vi "Iterate.vi"(6 "notifier in":refnum<notifier>, 8 "error in (no error)":errorcluster, 10 "Iterator Settings":T1={"Prepare timeout (ms)"=200, "Iterate timeout (ms)"=50, "Conclude timeout (ms)"=200, "Iterate period (ms)"=200, "Number of iterations"=5, "Stop Condition"=enum."None", "Time before stop (ms)"=5, "Prepare Msg"=refnum, "Iterate Msg"=refnum, "Conclude Msg"=refnum, "Error Handler"=refnum}, 11 "Caller Enqueuer in":refnum<class "Message Enqueuer.lvclass">) -> (0 "error out":errorcluster, 3 "Caller Enqueuer out":refnum<class "Message Enqueuer.lvclass">)   [LabVIEW 2017, in "Iterator Actor.lvlib" / "Iterator Actor.lvclass"]
doc: "Iteratively calls the Iterate method of the Client. \nStops the iterations either by receiving the Stop signal, or by any of predefined Stop conditions."
uses:
  Iterator Actor.lvclass
  Iterator Settings.ctl
  Iterator Actor Abstract Messages/Iterator Reply Msg/Iterator Reply Msg.lvclass
  C:/Program Files (x86)/National Instruments/LabVIEW 2017/vi.lib/ActorFramework/Message/Message.lvclass
  Iterator Actor Abstract Messages/Iterator Report Error Msg/Iterator Report Error Msg.lvclass
  Stop Condition.ctl
  <vilib>/ActorFramework/Message Enqueuer/Message Enqueuer.lvclass
  Iterator Actor Abstract Messages/Iterator Reply Msg/Iterator Reply Msg.lvclass/Iterator Reply Msg.ctl
  <vilib>/ActorFramework/Message Enqueuer/Message Enqueuer.lvclass/Message Enqueuer.ctl
  Iterator Errors.ctl
  <vilib>/ActorFramework/Message Enqueuer/Enqueue.vi
  <vilib>/ActorFramework/Message Priority Queue/Priority Enqueue.vi
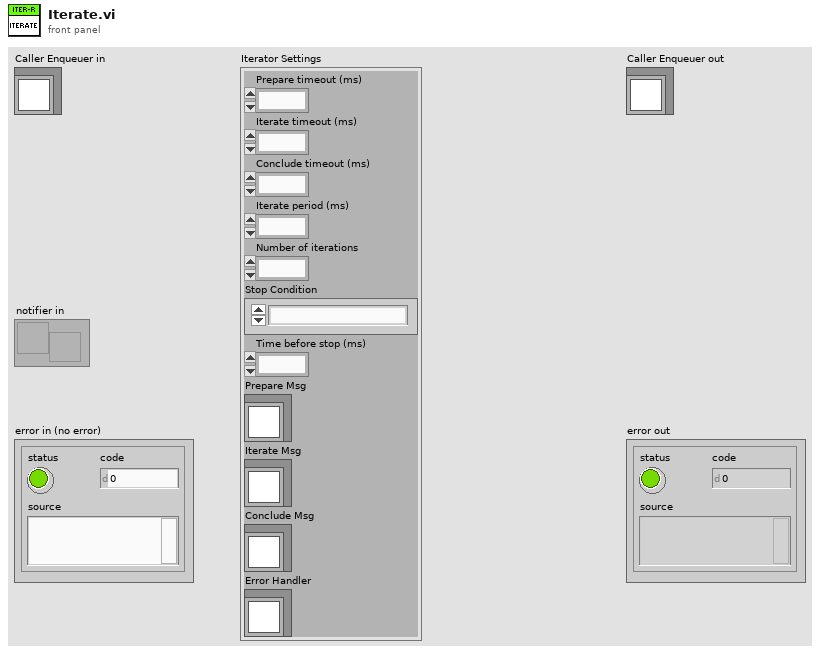
[diagram p1: front panel]
types:
  T1 = typedef "Iterator Actor.lvlib/Iterator Actor.lvclass/Iterator Settings.ctl" = cluster{"Prepare timeout (ms)":i32, "Iterate timeout (ms)":i32, "Conclude timeout (ms)":i32, "Iterate period (ms)":i32, "Number of iterations":i32, "Stop Condition":T2, "Time before stop (ms)":i32, "Prepare Msg":refnum<class "Iterator Reply Msg.lvclass">, "Iterate Msg":refnum<class "Iterator Reply Msg.lvclass">, "Conclude Msg":refnum<class "Iterator Reply Msg.lvclass">, "Error Handler":refnum<class "Iterator Report Error Msg.lvclass">}
  T2 = typedef "Iterator Actor.lvlib/Iterator Actor.lvclass/Stop Condition.ctl" = enum16{"None", "Number of Iterations", "Time Elapsed", "Iteration Result"}
  T3 = typedef "Iterator Actor.lvlib/Iterator Actor.lvclass/Iterator Errors.ctl" = enum16{"Input parameters are not valid", "Preparation call timed out", "Iteration call timed out", "Conclusion call timed out"}
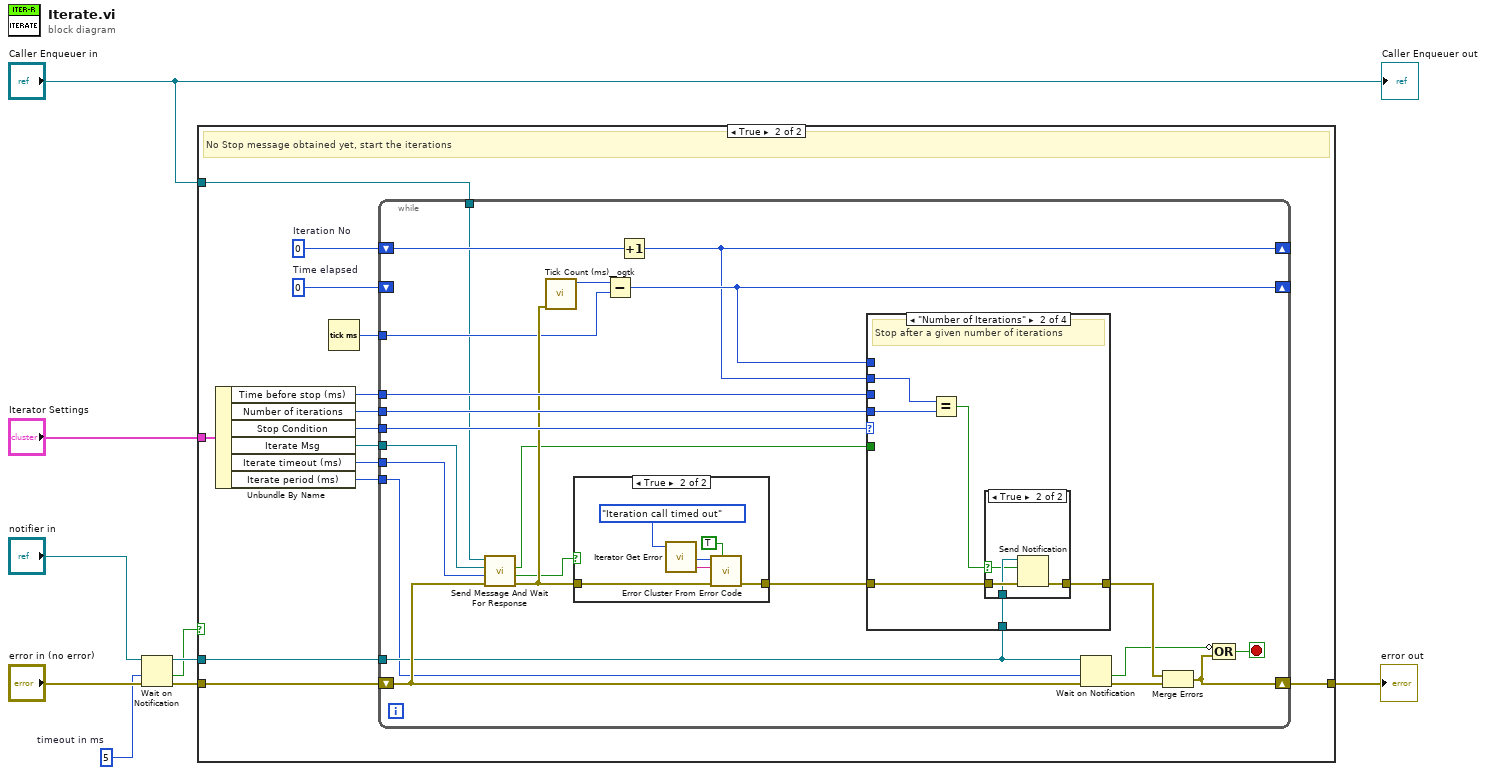
[diagram p0: block diagram]
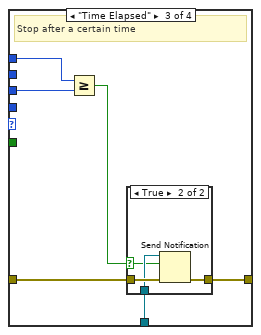
[diagram p5: hidden frame]
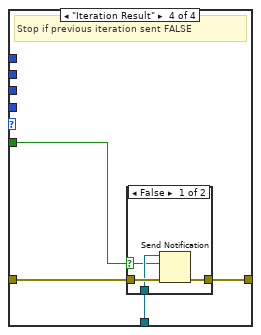
[diagram p7: hidden frame]
diagram:
  w1 = 5  # timeout in ms
  n1 = Wait on Notification(notifier="notifier in", timeout in ms (-1)=w1, error in (no error)="error in (no error)") -> (notifier out=w3:refnum<notifier>, timed out?=w2:bool, error out=w5:errorcluster)  [unwired: 1 in, 1 out]
  n2 = case shown="True" w2 {
    tunnel: "Iterator Settings" -> [_ w18]
    tunnel: "Caller Enqueuer in" -> [_ w15]
    tunnel: [w10 w13] -> w7
    tunnel: w5 -> [w10 w12]
    tunnel: w3 -> [_ w11]
    frame False {
      # "Stop message arrived before during the preparation. Do not proceed with iterations."
    }
    frame True {
      w14 = 0  # Iteration No
      w16 = u32 0  # Time elapsed
      # "No Stop message obtained yet, start the iterations"
      n3 = Unbundle By Name(w18) -> ("Time before stop (ms)"=w19:i32, "Number of iterations"=w20:i32, "Stop Condition"=w21:T2, "Iterate Msg"=w22:refnum<class "Iterator Reply Msg.lvclass">, "Iterate timeout (ms)"=w23:i32, "Iterate period (ms)"=w24:i32)
      n4 = Tick Count (ms)() -> (millisecond timer value=w17:u32)
      n5 = while {
        tunnel: w22 -> [w47]
        tunnel: w23 -> [w46]
        tunnel: w24 -> [w26]
        shift-right: [w27] -> w13
        shift-left: w12 -> [w29]
        shift-right: [w32] -> _
        shift-left: w14 -> [w42]
        shift-right: [w33] -> _
        shift-left: w16 -> [_]
        tunnel: w21 -> [w43]
        tunnel: w20 -> [w41]
        tunnel: w19 -> [w40]
        tunnel: w17 -> [w35]
        tunnel: w15 -> [w31]
        tunnel: w11 -> [w28]
        stop <- w39 stop-if-true
        n6 = call "Send Message And Wait For Response.vi"("error in (no error)"=w29, "timeout in ms (-1)"=w46, "Original Message"=w47, "Message Enqueuer in"=w31) -> ("error out"=w37:errorcluster, "timed out?"=w34:bool, "Reply"=w30:bool)  [unwired: 4 in, 1 out]
        n7 = call <userlib>:"Tick Count (ms)__ogtk.vi"("error in (no error)"=w37) -> ("millisecond timer value"=w36:u32)  [unwired: 9 in, 1 out]
        n8 = case shown="True" w34 {
          tunnel: w37 -> [w80 w83]
          tunnel: [w80 w82] -> w38
          frame False {
          }
          frame True {
            n9 = call "Iterator Get Error.vi"("Error"=Iterator_Errors."Iteration call timed out") -> ("source"=w85:string, "code"=w84:i32)  [unwired: 2 in, 1 out]
            n10 = call <vilib>:"Error Cluster From Error Code.vi"("show call chain? (False)"=TRUE ("is warning? (False)"), "error in (no error)"=w83, "error message (\"\")"=w85, "error code (0)"=w84) -> ("error out"=w82:errorcluster)  [unwired: 5 in]
          }
        }
        n11 = Subtract(x=w36, y=w35) -> (x-y=w33:u32)
        n12 = Increment(x=w42) -> (x+1=w32:i32)
        n13 = case shown="\"Number of Iterations\"" w43 {
          tunnel: w38 -> [w48 w51 w65 w71]
          tunnel: [w48 w50 w64 w73] -> w44
          tunnel: w28 -> [_ w54 w63 w72]
          tunnel: w41 -> [_ w53 _ _]
          tunnel: w40 -> [_ _ w62 _]
          tunnel: w33 -> [_ _ w60 _]
          tunnel: w32 -> [_ w49 _ _]
          tunnel: w30 -> [_ _ _ w74]
          frame "None", Default {
            # "No stop conditions (only external)"
          }
          frame "Number of Iterations" {
            # "Stop after a given number of iterations"
            n14 = Equal?(x=w49, y=w53) -> (x = y?=w52:bool)
            n15 = case shown="True" w52 {
              selector: w52 -> [_ w56]
              tunnel: w54 -> [_ w57]
              tunnel: w51 -> [w55 w59]
              tunnel: [w55 w58] -> w50
              frame False {
              }
              frame True {
                n16 = Send Notification(notification=w56, notifier=w57, error in (no error)=w59) -> (error out=w58:errorcluster)  [unwired: 1 out]
              }
            }
          }
          frame "Time Elapsed" {
            # "Stop after a certain time"
            n17 = Greater Or Equal?(x=w60, y=w62) -> (x >= y?=w61:bool)
            n18 = case shown="True" w61 {
              selector: w61 -> [_ w67]
              tunnel: w63 -> [_ w68]
              tunnel: w65 -> [w66 w70]
              tunnel: [w66 w69] -> w64
              frame False {
              }
              frame True {
                n19 = Send Notification(notification=w67, notifier=w68, error in (no error)=w70) -> (error out=w69:errorcluster)  [unwired: 1 out]
              }
            }
          }
          frame "Iteration Result" {
            # "Stop if previous iteration sent FALSE"
            n20 = case shown="False" w74 {
              selector: w74 -> [w75 _]
              tunnel: w72 -> [w76 _]
              tunnel: w71 -> [w78 w79]
              tunnel: [w77 w79] -> w73
              frame False {
                n21 = Send Notification(notification=w75, notifier=w76, error in (no error)=w78) -> (error out=w77:errorcluster)  [unwired: 1 out]
              }
              frame True {
              }
            }
          }
        }
        n22 = Wait on Notification(notifier=w28, timeout in ms (-1)=w26, error in (no error)=w29) -> (timed out?=w25:bool, error out=w45:errorcluster)  [unwired: 1 in, 2 out]
        n23 = Merge Errors(w44, w45) -> (w27:errorcluster)
        n24 = Compound Arithmetic op=OR(invert w25, w27) -> (w39:bool)
      }
    }
  }
  "error out" <- w7
  "Caller Enqueuer out" <- "Caller Enqueuer in"
